vi "dl950_wave.vi"() -> ()   [LabVIEW 2019]
uses:
  <instrlib>/Yokogawa DL950 Series/Yokogawa DL950 Series.lvlib
panel:
  in  "Record Length (0: 10k)":i32(ring) items=["10k", "25k", "50k", "100k", "250k", "500k", "1M", "2.5M", "5M", "10M", "25M", "50M", "100M", "250M", "500M", "1G", "2G", "4G", "5G", "10G", "20G", "50G"]
  in  "Count (0: Infinity)":u32
  in  "Acquisition Mode (0: Normal)":i32(ring) items=["Normal", "Average", "Envelope"]
  in  "VISA resource name":refnum<visa-resource-name>
  out "error out 2":errorcluster
  in  "error in (no error) 2":errorcluster
  out "VISA resource name out":refnum<visa-resource-name>
  in  "Time Division (12: 1ms)":i32(ring)=12 items=["100ns", "200ns", "500ns", "1us", "2us", "5us", "10us", "20us", "50us", "100us", "200us", "500us", "1ms", "2ms", "5ms", "10ms", "20ms", "50ms", "100ms", "200ms", "500ms", "1s", "2s", "3s", "4s", "5s", "6s", "10s", "20s", "30s", "1min", "2min", "3min", "4min", "5min", "6min", "10min", "12min", "30min", "1hour", "2hour", "3hour", "4hour", "5hour", "6hour", "8hour", "10hour", "12hour", "1day", "2day", "3day", "4day", "5day"]
  in  "VISA resource name 2":refnum<visa-resource-name>
  in  "ID Query (True)":bool=TRUE
  out "read buffer":string
  in  "error in (no error)":errorcluster
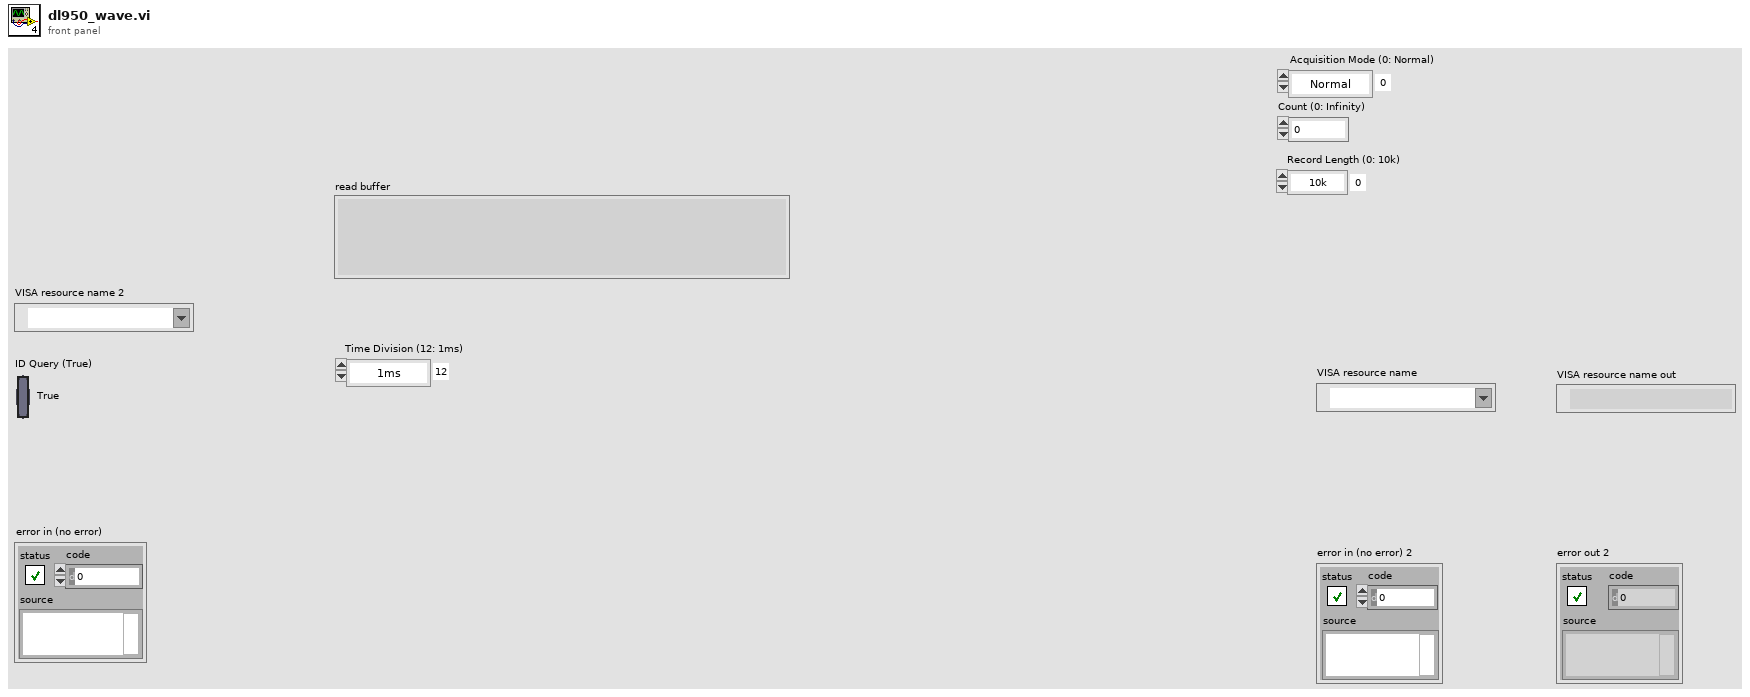
[diagram p1: front panel]
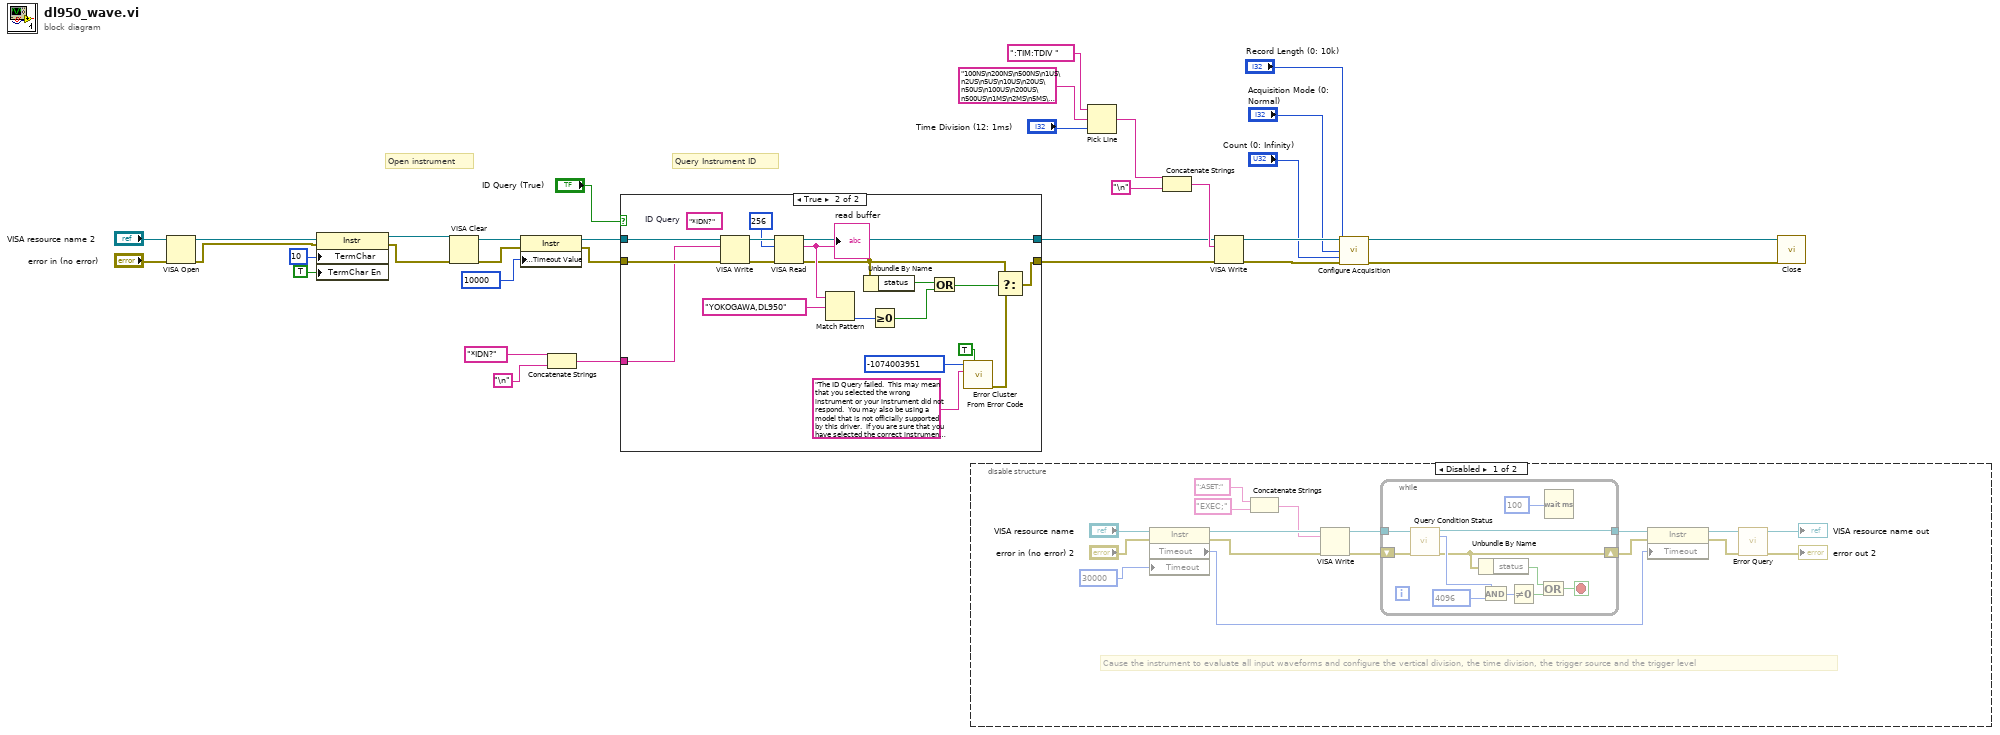
[diagram p0: block diagram]
diagram:
  # "Query Instrument ID"
  # "Open instrument"
  n1 = VISA Open ("VISAオープン")(error in (no error)="error in (no error)", VISA resource name="VISA resource name 2") -> (VISA resource name=w19:refnum<visa-resource-name>, error out=w18:errorcluster)  [unwired: 3 in]
  n2 = property class="Instr"(reference=w19, error in=w18, "TermChar"=u8 10 ("Message Based Settings:Termination Character"), "TermChar En"=TRUE ("Message Based Settings:Termination Character Enable")) -> (reference out=w17:refnum<visa-resource-name>, error out=w16:errorcluster)
  n3 = VISA Clear ("VISAクリア")(VISA resource name=w17, error in (no error)=w16) -> (VISA resource name out=w28:refnum<visa-resource-name>, error out=w27:errorcluster)
  n4 = property on="プロパティノード" class="Instr"(reference=w28, error in=w27, "General Settings:Timeout Value"=u32 10000) -> (reference out=w26:refnum<visa-resource-name>, error out=w25:errorcluster)
  n5 = Concatenate Strings("*IDN?" ("Command"), "\n") -> (w22:string)
  n6 = case "ケースストラクチャ" shown="True" "ID Query (True)" {
    tunnel: [w33 w53] -> w9
    tunnel: [w34 w50] -> w10
    tunnel: w26 -> [w34 w51]
    tunnel: w25 -> [w33 w52]
    tunnel: w22 -> [_ w35]
    frame False {
    }
    frame True {
      (unwired) "*IDN?"  # ID Query
      n7 = VISA Write ("VISA書き込み")(VISA resource name=w51, write buffer=w35, error in (no error)=w52) -> (VISA resource name out=w48:refnum<visa-resource-name>, error out=w47:errorcluster)  [unwired: 1 out]
      n8 = VISA Read ("VISA読み取り")(VISA resource name=w48, byte count=u32 256, error in (no error)=w47) -> (VISA resource name out=w50:refnum<visa-resource-name>, read buffer=w49:string, error out=w39:errorcluster)  [unwired: 1 out]
      "read buffer" <- w49
      n9 = Match Pattern ("パターンで一致")(string=w49, regular expression="YOKOGAWA,DL950") -> (offset past match=w40:i32)  [unwired: 1 in, 3 out]
      n10 = Unbundle By Name ("名前でバンドル解除")(w39) -> ("status"=w37:bool)
      n11 = Greater Or Equal To 0? ("0Èã?")(x=w40) -> (x >= 0?=w36:bool)
      n12 = Or(x=w37, y=w36) -> (x .or. y?=w38:bool)
      n13 = call <vilib>:"Error Cluster From Error Code.vi"("show call chain? (False)"=TRUE, "error message (\"\")"="The ID Query failed.  This may mean that you selected the wrong instrument or your instrument did not respond.  You may also be using a model that is not officially supported by this driver.  If you are sure that you have selected the correct instrument and it is responding, try disabling the ID Query." ("Source (VI Name)"), "error code (0)"=-1074003951 ("Code")) -> ("error out"=w44:errorcluster)  [unwired: 6 in]
      n14 = Select ("‘I‘ð")(t=w39, s=w38, f=w44) -> (s? t:f=w53:errorcluster)
    }
  }
  n15 = disable-structure shown="Disabled" {
    frame Disabled {
      # "Cause the instrument to evaluate all input waveforms and configure the vertical division, the time division, the trigger source and the trigger level"
      n16 = property class="Instr"(reference="VISA resource name", error in="error in (no error) 2", "Timeout"=u32 30000 ("General Settings:Timeout Value")) -> (reference out=w66:refnum<visa-resource-name>, error out=w55:errorcluster, "Timeout"=w64:u32)
      n17 = Concatenate Strings ("•¶Žš—ñ˜AŒ‹")(":ASET:", "EXEC;") -> (w57:string)
      n18 = VISA Write ("VISA書き込み")(VISA resource name=w66, write buffer=w57, error in (no error)=w55) -> (VISA resource name out=w61:refnum<visa-resource-name>, error out=w60:errorcluster)  [unwired: 1 out]
      n19 = while {
        tunnel: w61 -> [w76]
        tunnel: [w74] -> w59
        shift-right: [w71] -> w58
        shift-left: w60 -> [w75]
        stop <- w78 stop-if-true
        n20 = call <instrlib>:"Query Condition Status.vi"("VISA resource name"=w76, "error in (no error)"=w75) -> ("VISA resource name out"=w74:refnum<visa-resource-name>, "Condition Status"=w73:i32, "error out"=w71:errorcluster)  [unwired: 11 in]
        n21 = Unbundle By Name(w71) -> ("status"=w79:bool)
        n22 = And(x=w73, y=4096) -> (x .and. y?=w80:i32)
        n23 = Not Equal To 0?(x=w80) -> (x != 0?=w72:bool)
        n24 = Or(x=w79, y=w72) -> (x .or. y?=w78:bool)
        n25 = Wait (ms)(milliseconds to wait=u32 100) -> ()  [unwired: 1 out]
      }
      n26 = property class="Instr"(reference=w59, error in=w58, "Timeout"=w64) -> (reference out=w63:refnum<visa-resource-name>, error out=w62:errorcluster)
      n27 = call <instrlib>:"Error Query.vi"("error in (no error)"=w62, "VISA resource name"=w63) -> ("error out"=→"error out 2":errorcluster, "VISA resource name out"=→"VISA resource name out":refnum<visa-resource-name>)  [unwired: 6 in, 2 out]
    }
    frame Enabled {
    }
  }
  n28 = Pick Line ("ライン選択")(string ("")=":TIM:TDIV ", multi-line string="100NS\n200NS\n500NS\n1US\n2US\n5US\n10US\n20US\n50US\n100US\n200US\n500US\n1MS\n2MS\n5MS\n10MS\n20MS\n50MS\n100MS\n200MS\n500MS\n1S\n2S\n3S\n4S\n5S\n6S\n10S\n20S\n30S\n60S\n120S\n180S\n240S\n300S\n360S\n600S\n720S\n1800S\nHOUR1\nHOUR2\nHOUR3\nHOUR4\nHOUR5\nHOUR6\nHOUR8\nHOUR10\nHOUR12\nDAY1\nDAY2\nDAY3\nDAY4\nDAY5", line index="Time Division (12: 1ms)") -> (output string=w12:string)
  n29 = Concatenate Strings(w12, "\n") -> (w11:string)
  n30 = VISA Write ("VISA書き込み")(VISA resource name=w10, write buffer=w11, error in (no error)=w9) -> (VISA resource name out=w7:refnum<visa-resource-name>, error out=w6:errorcluster)  [unwired: 1 out]
  n31 = call <instrlib>:"Configure Acquisition.vi"("VISA resource name"=w7, "Record Length (0: 10k)"="Record Length (0: 10k)", "Acquisition Mode (0: Normal)"="Acquisition Mode (0: Normal)", "Count (0: Infinity)"="Count (0: Infinity)", "error in (no error)"=w6) -> ("VISA resource name out"=w2:refnum<visa-resource-name>, "error out"=w1:errorcluster)  [unwired: 9 in]
  n32 = call <instrlib>:"Close.vi"("error in (no error)"=w1, "VISA resource name"=w2) -> ()  [unwired: 9 in, 1 out]
